vi "Create Information Channels.vi"(7 "error in (no error)":errorcluster, 10 "Node Ptr":u64 format="%.0x") -> (0 "error out":errorcluster)   [LabVIEW 2023, in "Protection and Counter Addon System Explorer.lvlib"]
uses:
  Protection and Counter Addon System Explorer.lvlib
  <vilib>/NI VeriStand/Custom Device API/Custom Device Item Ref.ctl
  <vilib>/NI VeriStand/Custom Device API/Custom Device API.lvlib
panel:
  out "Parent Ref out":T1 format="%.0x"
  in  "Tag":string
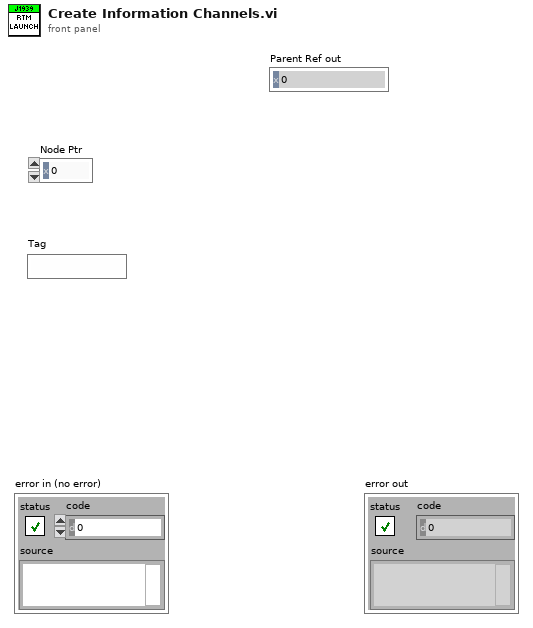
[diagram p1: front panel]
types:
  T1 = typedef "Custom Device API.lvlib/Custom Device Item Ref.ctl" = u64
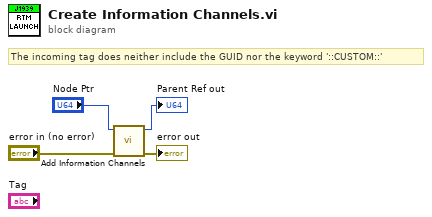
[diagram p0: block diagram]
diagram:
  # "The incoming tag does neither include the GUID nor the keyword '::CUSTOM::'"
  n1 = call "Add Information Channels.vi"("error in (no error)"="error in (no error)", "Node Ptr"="Node Ptr") -> ("error out"=→"error out":errorcluster, "Parent Ref out"=→"Parent Ref out":T1)  [unwired: 8 in]
